vi "WSVCAP SHL FPGA LL I2C Write Data Lines.vi"(0 "Write Bit (U64)":u64, 11 "error in (no error)":errorcluster, 13 "Socket Mask":u64 format="%012x", 14 "UUT Set (0/1)":u8) -> (15 "error out":errorcluster)   [LabVIEW 2012]
uses:
  WSVCAP SHL FPGA LL I2C Debug Global.vi
  <vilib>/eio/EIONode/EIONode.xnode
  <vilib>/rvi/eio/common/nirviEmuTemplateMethod_errors.vi
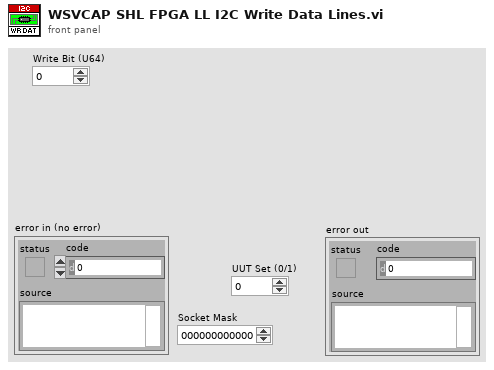
[diagram p1: front panel]
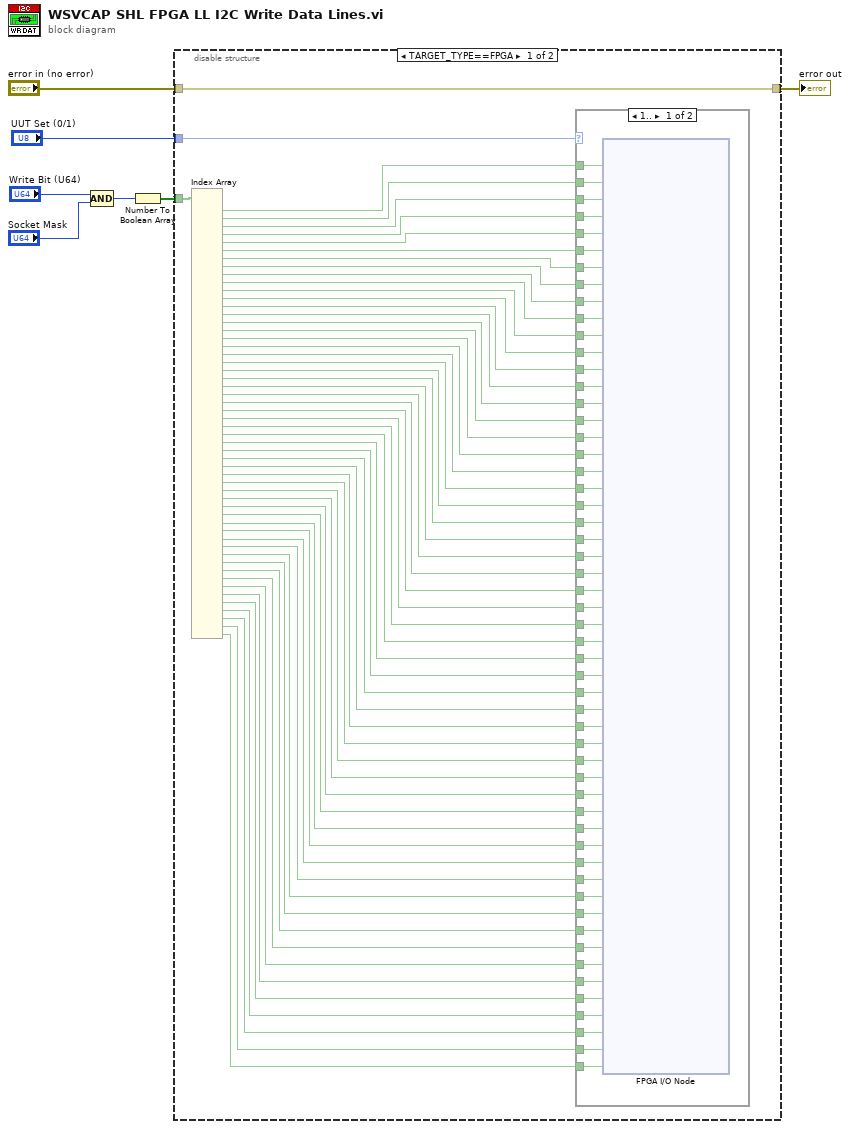
[diagram p0: block diagram]
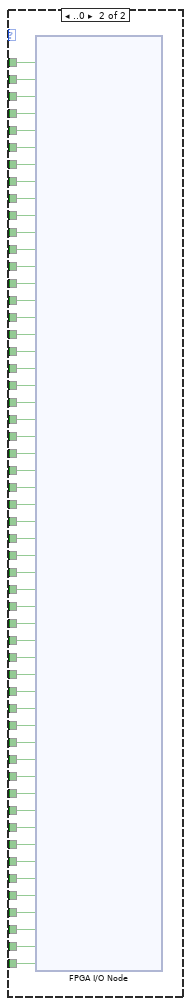
[diagram p2: hidden frame]
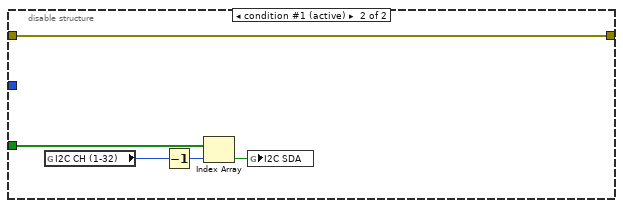
[diagram p3: hidden frame]
diagram:
  n1 = Compound Arithmetic op=AND("Write Bit (U64)", "Socket Mask") -> (w2:u64)
  n2 = Number To Boolean Array(number=w2) -> (Boolean array=w5:bool[])
  n3 = disable-structure shown="TARGET_TYPE==FPGA" {
    disable-tunnel: w5 -> [w48 w176]
    disable-tunnel: [w49 w177] -> w7
    disable-tunnel: "error in (no error)" -> [w49 w177]
    disable-tunnel: "UUT Set (0/1)" -> [w10 _]
    frame condition #0 {
      n4 = Index Array(array=w48) -> (element #1=w64:bool, element #2=w63:bool, element #3=w62:bool, element #4=w61:bool, element #5=w60:bool, element #6=w59:bool, element #7=w58:bool, element #8=w57:bool, element #9=w56:bool, element #10=w55:bool, element #11=w54:bool, element #12=w53:bool, element #13=w52:bool, element #14=w51:bool, element #15=w50:bool, element #16=w47:bool, element #17=w46:bool, element #18=w45:bool, element #19=w44:bool, element #20=w43:bool, element #21=w42:bool, element #22=w41:bool, element #23=w40:bool, element #24=w39:bool, element #25=w38:bool, element #26=w37:bool, element #27=w36:bool, element #28=w35:bool, element #29=w34:bool, element #30=w33:bool, element #31=w32:bool, element #32=w31:bool, element #33=w30:bool, element #34=w29:bool, element #35=w28:bool, element #36=w27:bool, element #37=w26:bool, element #38=w25:bool, element #39=w24:bool, element #40=w23:bool, element #41=w22:bool, element #42=w21:bool, element #43=w20:bool, element #44=w19:bool, element #45=w18:bool, element #46=w17:bool, element #47=w16:bool, element #48=w15:bool, element #49=w14:bool, element #50=w13:bool, element #51=w12:bool, element #52=w11:bool, element #53=w9:bool, element #54=w8:bool)  [unwired: 54 in]
      n5 = case shown="1.." w10 {
        tunnel: w64 -> [w118 w172]
        tunnel: w63 -> [w117 w171]
        tunnel: w62 -> [w116 w170]
        tunnel: w61 -> [w115 w169]
        tunnel: w60 -> [w114 w168]
        tunnel: w59 -> [w113 w167]
        tunnel: w58 -> [w112 w166]
        tunnel: w57 -> [w111 w165]
        tunnel: w56 -> [w110 w164]
        tunnel: w55 -> [w109 w163]
        tunnel: w54 -> [w108 w162]
        tunnel: w53 -> [w107 w161]
        tunnel: w52 -> [w106 w160]
        tunnel: w51 -> [w105 w159]
        tunnel: w50 -> [w104 w158]
        tunnel: w47 -> [w103 w157]
        tunnel: w46 -> [w102 w156]
        tunnel: w45 -> [w101 w155]
        tunnel: w44 -> [w100 w154]
        tunnel: w43 -> [w99 w153]
        tunnel: w42 -> [w98 w152]
        tunnel: w41 -> [w97 w151]
        tunnel: w40 -> [w96 w150]
        tunnel: w39 -> [w95 w149]
        tunnel: w38 -> [w94 w148]
        tunnel: w37 -> [w93 w147]
        tunnel: w36 -> [w92 w146]
        tunnel: w35 -> [w91 w145]
        tunnel: w34 -> [w90 w144]
        tunnel: w33 -> [w89 w143]
        tunnel: w32 -> [w88 w142]
        tunnel: w31 -> [w87 w141]
        tunnel: w30 -> [w86 w140]
        tunnel: w29 -> [w85 w139]
        tunnel: w28 -> [w84 w138]
        tunnel: w27 -> [w83 w137]
        tunnel: w26 -> [w82 w136]
        tunnel: w25 -> [w81 w135]
        tunnel: w24 -> [w80 w134]
        tunnel: w23 -> [w79 w133]
        tunnel: w22 -> [w78 w132]
        tunnel: w21 -> [w77 w131]
        tunnel: w20 -> [w76 w130]
        tunnel: w19 -> [w75 w129]
        tunnel: w18 -> [w74 w128]
        tunnel: w17 -> [w73 w127]
        tunnel: w16 -> [w72 w126]
        tunnel: w15 -> [w71 w125]
        tunnel: w14 -> [w70 w124]
        tunnel: w13 -> [w69 w123]
        tunnel: w12 -> [w68 w122]
        tunnel: w11 -> [w67 w121]
        tunnel: w9 -> [w66 w120]
        tunnel: w8 -> [w65 w119]
        frame 1.. {
          n6 = xnode "FPGA I/O Node"("I2C_SDA_C1_S19"=w118, "I2C_SDA_C1_S20"=w117, "I2C_SDA_C1_S21"=w116, "I2C_SDA_C1_S22"=w115, "I2C_SDA_C1_S23"=w114, "I2C_SDA_C1_S24"=w113, "I2C_SDA_C1_S25"=w112, "I2C_SDA_C1_S26"=w111, "I2C_SDA_C1_S27"=w110, "I2C_SDA_C1_S28"=w109, "I2C_SDA_C1_S29"=w108, "I2C_SDA_C1_S30"=w107, "I2C_SDA_C1_S31"=w106, "I2C_SDA_C1_S32"=w105, "I2C_SDA_C1_S33"=w104, "I2C_SDA_C1_S34"=w103, "I2C_SDA_C1_S35"=w102, "I2C_SDA_C1_S36"=w101, "I2C_SDA_C2_S19"=w100, "I2C_SDA_C2_S20"=w99, "I2C_SDA_C2_S21"=w98, "I2C_SDA_C2_S22"=w97, "I2C_SDA_C2_S23"=w96, "I2C_SDA_C2_S24"=w95, "I2C_SDA_C2_S25"=w94, "I2C_SDA_C2_S26"=w93, "I2C_SDA_C2_S27"=w92, "I2C_SDA_C2_S28"=w91, "I2C_SDA_C2_S29"=w90, "I2C_SDA_C2_S30"=w89, "I2C_SDA_C2_S31"=w88, "I2C_SDA_C2_S32"=w87, "I2C_SDA_C2_S33"=w86, "I2C_SDA_C2_S34"=w85, "I2C_SDA_C2_S35"=w84, "I2C_SDA_C2_S36"=w83, "I2C_SDA_C3_S19"=w82, "I2C_SDA_C3_S20"=w81, "I2C_SDA_C3_S21"=w80, "I2C_SDA_C3_S22"=w79, "I2C_SDA_C3_S23"=w78, "I2C_SDA_C3_S24"=w77, "I2C_SDA_C3-S25"=w76, "I2C_SDA_C3_S26"=w75, "I2C_SDA_C3_S27"=w74, "I2C_SDA_C3_S28"=w73, "I2C_SDA_C3_S29"=w72, "I2C_SDA_C3_S30"=w71, "I2C_SDA_C3_S31"=w70, "I2C_SDA_C3_S32"=w69, "I2C_SDA_C3_S33"=w68, "I2C_SDA_C3_S34"=w67, "I2C_SDA_C3_S35"=w66, "I2C_SDA_C3_S36"=w65) -> ()  [unwired: 54 in, 54 out]
        }
        frame ..0 {
          n7 = xnode "FPGA I/O Node"("I2C_SDA_C1_S1"=w172, "I2C_SDA_C1_S2"=w171, "I2C_SDA_C1_S3"=w170, "I2C_SDA_C1_S4"=w169, "I2C_SDA_C1_S5"=w168, "I2C_SDA_C1_S6"=w167, "I2C_SDA_C1_S7"=w166, "I2C_SDA_C1_S8"=w165, "I2C_SDA_C1_S9"=w164, "I2C_SDA_C1_S10"=w163, "I2C_SDA_C1_S11"=w162, "I2C_SDA_C1_S12"=w161, "I2C_SDA_C1_S13"=w160, "I2C_SDA_C1_S14"=w159, "I2C_SDA_C1_S15"=w158, "I2C_SDA_C1_S16"=w157, "I2C_SDA_C1_S17"=w156, "I2C_SDA_C1_S18"=w155, "I2C_SDA_C2_S1"=w154, "I2C_SDA_C2_S2"=w153, "I2C_SDA_C2_S3"=w152, "I2C_SDA_C2_S4"=w151, "I2C_SDA_C2_S5"=w150, "I2C_SDA_C2_S6"=w149, "I2C_SDA_C2_S7"=w148, "I2C_SDA_C2_S8"=w147, "I2C_SDA_C2_S9"=w146, "I2C_SDA_C2_S10"=w145, "I2C_SDA_C2_S11"=w144, "I2C_SDA_C2_S12"=w143, "I2C_SDA_C2_S13"=w142, "I2C_SDA_C2_S14"=w141, "I2C_SDA_C2_S15"=w140, "I2C_SDA_C2_S16"=w139, "I2C_SDA_C2_S17"=w138, "I2C_SDA_C2_S18"=w137, "I2C_SDA_C3_S1"=w136, "I2C_SDA_C3_S2"=w135, "I2C_SDA_C3_S3"=w134, "I2C_SDA_C3_S4"=w133, "I2C_SDA_C3_S5"=w132, "I2C_SDA_C3_S6"=w131, "I2C_SDA_C3_S7"=w130, "I2C_SDA_C3_S8"=w129, "I2C_SDA_C3_S9"=w128, "I2C_SDA_C3_S10"=w127, "I2C_SDA_C3_S11"=w126, "I2C_SDA_C3_S12"=w125, "I2C_SDA_C3_S13"=w124, "I2C_SDA_C3_S14"=w123, "I2C_SDA_C3_S15"=w122, "I2C_SDA_C3_S16"=w121, "I2C_SDA_C3_S17"=w120, "I2C_SDA_C3_S18"=w119) -> ()  [unwired: 54 in, 54 out]
        }
      }
    }
    frame condition #1 (active) {
      n8 = global read "WSVCAP SHL FPGA LL I2C Debug Global.vi" "I2C CH (1-32)"() -> (w175:i32)
      n9 = Decrement(x=w175) -> (x-1=w173:i32)
      n10 = Index Array(array=w176, index=w173) -> (element=w174:bool)
      n11 = global write "WSVCAP SHL FPGA LL I2C Debug Global.vi" "I2C SDA"(w174) -> ()
    }
  }
  "error out" <- w7
